vi "Pre Launch Init.vi"(11 "Line Tracker in":refnum<class "Line Tracker.lvclass">) -> (0 "error out":errorcluster, 3 "Line Tracker out":refnum<class "Line Tracker.lvclass">)   [LabVIEW 2026, in "Line Tracker.lvlib" / "Line Tracker.lvclass"]
doc: "<p>(<strong>Filename</strong>: <span class=\"dnl\">Actor Framework.lvlib:Actor.lvclass:Pre Launch Init.vi</span>)</p>\n<p>Defines behavior that occurs after the <a href=\"nihelplauncher://docs/csh?context=lvcore_lvcomm_af_launch_nested_actor\">Launch Nested Actor</a> method is invoked but before the actor's Actor Core method begins running.</p>\n<p>By default, this method does nothing. A descendant class may override it to define behavior.</p>"
uses:
  Line Tracker.lvclass
  Line Tracker.lvclass/Line Tracker.ctl
  CTI-Grove/Examples/Sourcecode/cti-drivers-lv-visa-simple/Examples/Driver/CTIPicoVISA.lvlib
  CTI-Grove/Examples/Sourcecode/cti-drivers-lv-visa-simple/Examples/Driver/Public/Digital Direction.ctl
  <vilib>/ActorFramework/Actor/Actor.lvclass
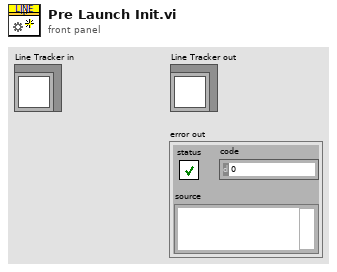
[diagram p1: front panel]
types:
  T1 = typedef "CTIPicoVISA.lvlib/Digital Direction.ctl" = enum16{"In", "Out"}
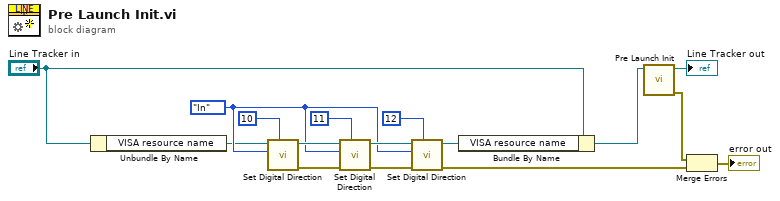
[diagram p0: block diagram]
diagram:
  w8 = Digital_Direction."In" ("Direction")
  n1 = Unbundle By Name("Line Tracker in") -> ("VISA resource name"=w5:refnum<visa-resource-name>)
  n2 = call "Set Digital Direction.vi"("GPIO"=10, "Direction"=w8, "VISA resource name in"=w5) -> ("error out"=w12:errorcluster, "VISA resource name"=w13:refnum<visa-resource-name>)  [unwired: 7 in]
  n3 = call "Set Digital Direction.vi"("GPIO"=11, "error in (no error)"=w12, "Direction"=w8, "VISA resource name in"=w13) -> ("error out"=w11:errorcluster, "VISA resource name"=w9:refnum<visa-resource-name>)  [unwired: 6 in]
  n4 = call "Set Digital Direction.vi"("GPIO"=12, "error in (no error)"=w11, "Direction"=w8, "VISA resource name in"=w9) -> ("error out"=w3:errorcluster, "VISA resource name"=w1:refnum<visa-resource-name>)  [unwired: 6 in]
  n5 = Bundle By Name(cluster="Line Tracker in", "VISA resource name"=w1) -> (w2:refnum<class "Line Tracker.lvclass">)
  n6 = call-parent "Pre Launch Init.vi"("Actor in"=w2) -> ("error out"=w16:errorcluster, "Actor out"=→"Line Tracker out":refnum<class "Line Tracker.lvclass">)  [unwired: 9 in]
  n7 = Merge Errors(w16, w3) -> (→"error out":errorcluster)
